vi "FunctionGeneratorMatrix_New.vi"(9 "Columns":i32=1, 11 "Rows":i32=1) -> (3 "FUNCTION_GENERATOR_MATRIX":T1)   [LabVIEW 2019, in "Trajectory_Library.lvlib"]
doc: "Function generator matrix ( Interpolating Tree Maps) are used to get values at points that are not defined by making a guess from points that are defined. This uses linear interpolation. This type returns a Y matrix as a function of a provided double X value. \n\nInputs:\n -- Rows -- Number of rows in the Y matrix\n -- Columns -- Number of columns in the Y matrix. \n\nOutputs:\n - Function Generator Matrix -- Created data cluster"
uses:
  Trajectory_Library.lvlib
  FUNCTION_GENERATOR_MATRIX.ctl
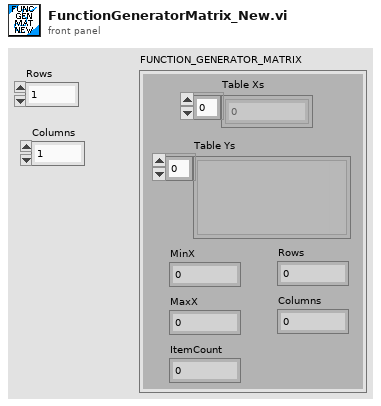
[diagram p1: front panel]
types:
  T1 = typedef "Trajectory_Library.lvlib/FUNCTION_GENERATOR_MATRIX.ctl" = cluster{"Table Xs":dbl[], "Table Ys":variant[], "MinX":dbl, "MaxX":dbl, "ItemCount":i32, "Rows":i32, "Columns":i32}
  T2 = typedef "NI_Matrix.lvlib/RealMatrix.ctl" = dbl[][]
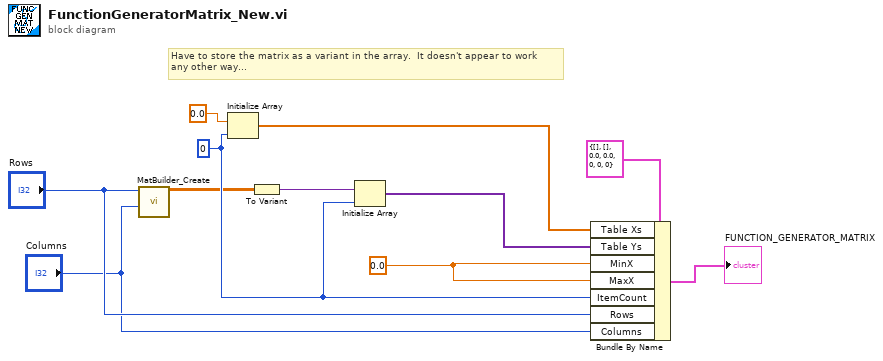
[diagram p0: block diagram]
diagram:
  w8 = 0.0 ("X")
  w6 = 0 ("dimension size")
  # "Have to store the matrix as a variant in the array.  It doesn't appear to work\nany other way..."
  n1 = call "MatBuilder_Create.vi"("Columns"="Columns", "Rows"="Rows") -> ("output matrix"=w5:T2)  [unwired: 9 in]
  n2 = Initialize Array(0.0 ("element"), w6) -> (w9:dbl[])
  n3 = To Variant(anything=w5) -> (Variant=w4:variant)
  n4 = Initialize Array(w4, w6) -> (w3:variant[])
  n5 = Bundle By Name(cluster=T1 {"Table Xs"=[], "Table Ys"=[], "MinX"=0.0, "MaxX"=0.0, "ItemCount"=0, "Rows"=0, "Columns"=0} ("FUNCTION_GENERATOR_MATRIX"), "Table Xs"=w9, "Table Ys"=w3, "MinX"=w8, "MaxX"=w8, "ItemCount"=w6, "Rows"="Rows", "Columns"="Columns") -> (→"FUNCTION_GENERATOR_MATRIX":T1)
